vi "Enable Timers.vi"(0 "FPGA Ref":T6, 1 "Tank Data":T8 {"PS Actual (V):" format="%.2f"; "Temp1" format="%#_2g"; "Temp2" format="%#_2g"}, 2 "Tank CMDs":T7, 3 "App Config":T2={"Location"="", "Profiles Path"=path "", "Current Profile"="", "CA Number"="", "Cycles Completed"=0, "Controller Type:"=enum."Kuhnke", "Stagger Time (ms)"=0, "Tank 1 Fuel"="", "Tank 2 Fuel"="", "Serial Numbers"={"Position 1 SN"="", "Position 2 SN"="", "Poaition 3 SN"="", "Position 4 SN"="", "Position 5 SN"="", "Position 6 SN"=""}, "Pumps Present"={"Pump 1"=FALSE, "Pump 2"=FALSE, "Pump 3"=FALSE, "Pump 4"=FALSE, "Pump 5"=FALSE, "Pump 6"=FALSE}, "VoltCtrlRef"="", "VoltageSelect"=FALSE, "Watlow Present"=FALSE, "Temp 1"=0.0, "Temp 2"=0.0, "V_Run PI?"=FALSE, "Voltage Limits"={"V_Step"=1e-05, "V_CmdMax"=0.0, "V_CmdMin"=0.0}, "Voltage Far PI"={"V_FarSlew"=10.0, "V_FarKp"=0.0, "V_FarKi"=0.0}, "Voltage Mid PI"={"V_MidSlew"=10.0, "V_MidKp"=0.0, "V_MidKi"=0.0}, "Voltage Close PI"={"V_CloseSlew"=10.0, "V_CloseKp"=0.0, "V_CloseKi"=0.0}, "Voltage Scale"={"V_FFm"=0.0, "V_FFb"=0.0}, "Voltage Cutoffs"={"V_MidCutoff"=0.0, "V_CloseCutoff"=0.0}, "Pressure Scale"={"Pres_FFm"=1e-05, "Pres_FFb"=0.0}, "Temp Format"=0, "Temp Tolerance"=0.0, "Target Voltage"=0.0, "Target Pressure"=0.0, "Data Log Init"={"Data Path"=path "", "Data Log Rate (S/s)"=0, "AKLH Rate (Hours/S)"=0.0, "Sync Time Offset (min)"=0, "IP Last 3"=0, "WebDAV IP"=""}, "Email Handler IP"="", "ADC Check"=FALSE, "3 Pump Tank"=FALSE, "Cycle Threshold:"=3.0, "Cycle Pts to Avg:"=3, "Anomaly Threshold:"=3.0, "Normal Steps:"=3, "Step Threshold:"=3.0, "Network Drive IP"="", "Network Drive Password"="", "Bank 1 Offset"=0.0, "Bank 2 Offset"=0.0} {"Bank 2 Offset" min=0.0 max=999999.0 step=1.0; "Bank 1 Offset" min=0.0 max=999999.0 step=1.0; "Step Threshold:" min=0.0 max=999999.0 step=1.0; "Normal Steps:" max=999999 step=1; "Anomaly Threshold:" min=0.0 max=999999.0 step=1.0; "Cycle Pts to Avg:" max=999999 step=1; "Cycle Threshold:" min=0.0 max=999999.0 step=1.0}, 4 "Controller CMDs":dbl[](array[numeric]), 5 "Controller Config":T5, 6 "Run Profile":bool, 7 "Pumps Present":bool[](array[boolean])) -> (20 "In Spec":bool[](array[boolean]), 21 "Reset ADCs":bool)   [LabVIEW 2018]
uses:
  Controls/FPGA_Reference.ctl
  <vilib>/rvi/interface/nirviReadWriteControl/nirviReadWriteControl.xnode
  FPGA Bitfiles/LS_Durability_FPGA_9627.lvbitx
  <vilib>/rvi/errors/niLvFpgaMergeErrorWithErrorCode.vi
  <vilib>/rvi/errors/niLvFpgaAdjustHostInterfaceError.vi
  Controls/Tank Data.ctl
  Controls/Tank CMDs.ctl
  Type Defs/Controller Names.ctl
  Controls/Controller Config.ctl
  Type Defs/App Config.ctl
  Controls/Pump Data.ctl
  Data Logger/Data Log Init.ctl
panel:
  in  "Pump Data":T1={"Voltages"=[0.015201568603515625, 0.00335693359375, 0.003021240234375, 0.12260055541992188, 0.06085968017578125, 0.052234649658203125], "PumpCurrent"=[0.015201568603515625, 0.00335693359375, 0.003021240234375, 0.12260055541992188, 0.06085968017578125, 0.052234649658203125], "Speed"=[0.0, 0.0, 0.0, 0.0, 0.0, 0.0], "ControllerCurrent"=[0.015201568603515625, 0.00335693359375, 0.003021240234375, 0.12260055541992188, 0.06085968017578125, 0.052234649658203125], "Pressure"=[0.015201568603515625, 0.00335693359375, 0.003021240234375, 0.12260055541992188, 0.06085968017578125, 0.052234649658203125], "Flow"=[0.0, 0.0, 0.0, 0.125, 0.0625, 0.0625], "Elapsed Time (Display)"=[7.1, 7.1, 7.1, 458133.45, 458138.85000000003, 458126.75], "Avg Pressure"=0.0, "Avg Speed"=0.0, "Elapsed Time"=[4074.9003000000002, 4074.9003000000002, 4074.9003000000002, 4074.9003000000002, 4074.9003000000002, 4074.9003000000002]} {"Elapsed Time" format="%<%H:%M:%S>t"; "Elapsed Time (Display)" format="%<%H:%M:%S>t"; "Speed" format="%#_4f"; "ControllerCurrent" format="%#.1g"; "Pressure" format="%#.0f"; "Flow" format="%#.0f"; "PumpCurrent" format="%#.1g"; "Voltages" format="%#.0f"}
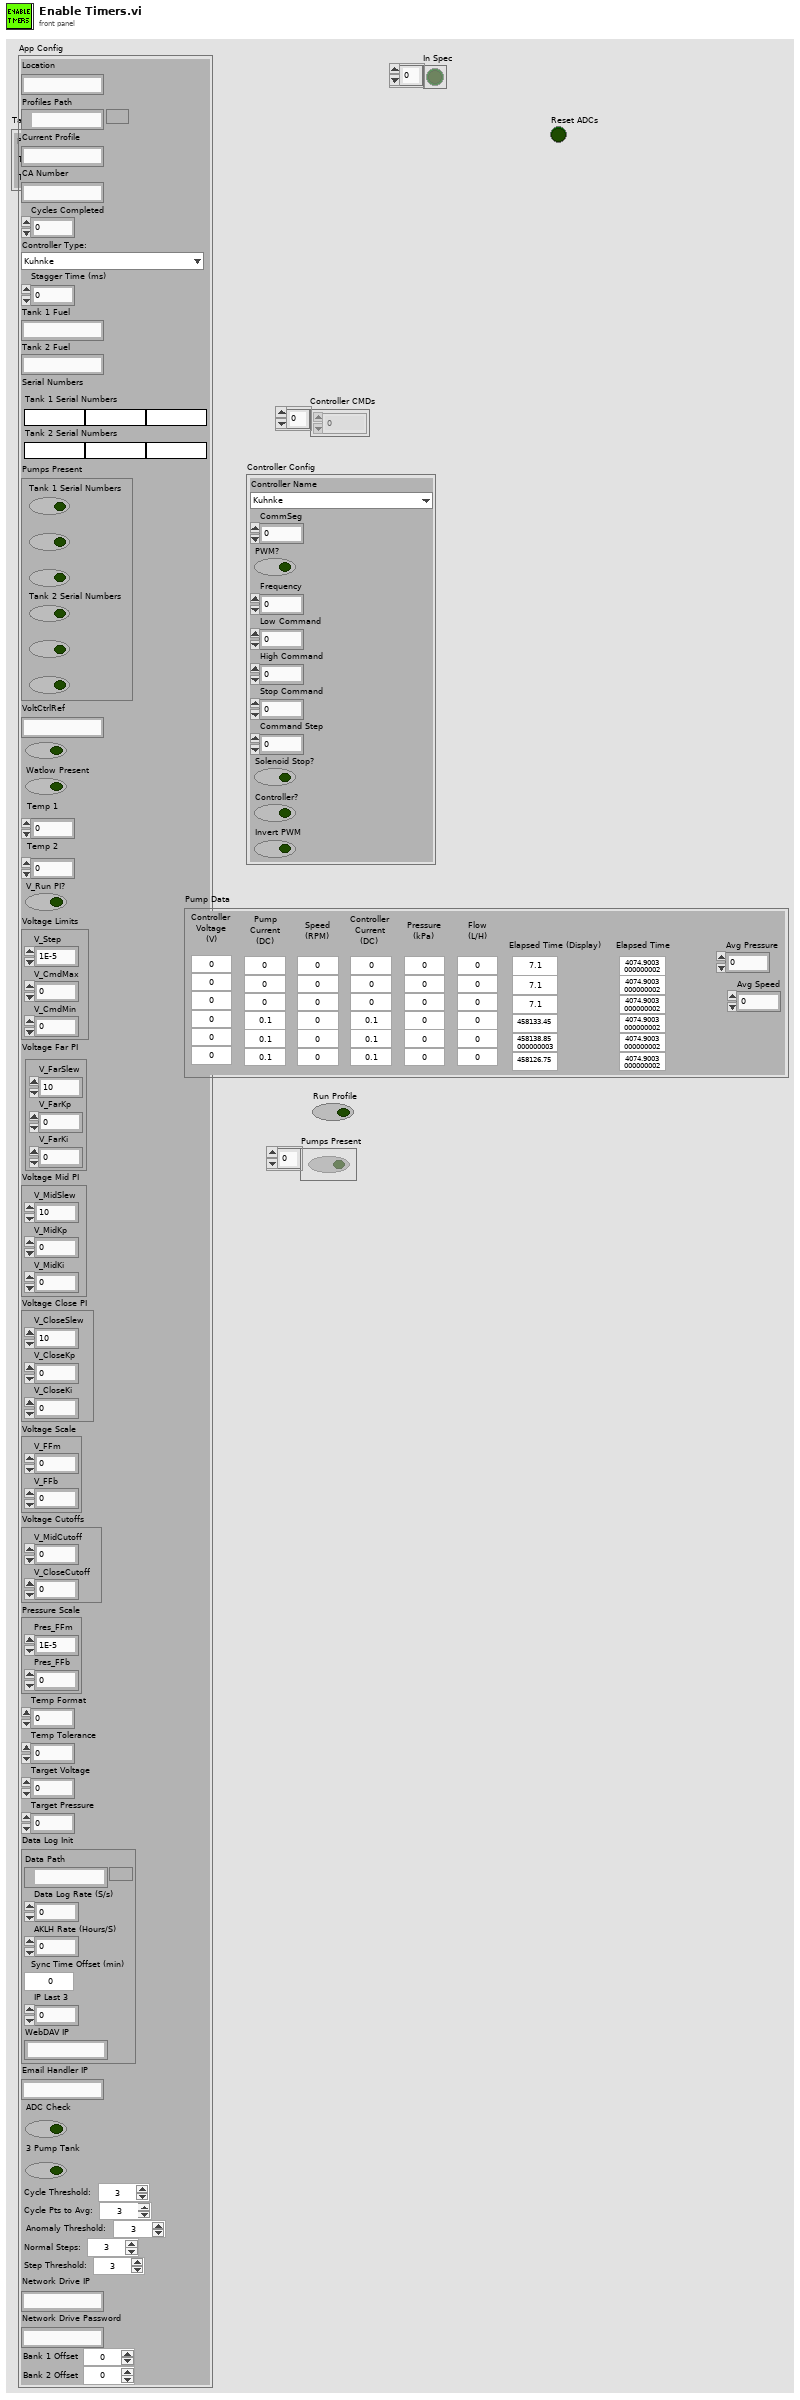
[diagram p1: front panel]
types:
  T1 = typedef "Pump Data.ctl" = cluster{"Voltages":dbl[], "PumpCurrent":dbl[], "Speed":dbl[], "ControllerCurrent":dbl[], "Pressure":dbl[], "Flow":dbl[], "Elapsed Time (Display)":dbl[], "Avg Pressure":dbl, "Avg Speed":dbl, "Elapsed Time":dbl[]}
  T2 = typedef "App Config.ctl" = cluster{"Location":string, "Profiles Path":path, "Current Profile":string, "CA Number":string, "Cycles Completed":u32, "Controller Type:":T3, "Stagger Time (ms)":i32, "Tank 1 Fuel":string, "Tank 2 Fuel":string, "Serial Numbers":cluster{"Position 1 SN":string, "Position 2 SN":string, "Poaition 3 SN":string, "Position 4 SN":string, "Position 5 SN":string, "Position 6 SN":string}, "Pumps Present":cluster{"Pump 1":bool, "Pump 2":bool, "Pump 3":bool, "Pump 4":bool, "Pump 5":bool, "Pump 6":bool}, "VoltCtrlRef":string, "VoltageSelect":bool, "Watlow Present":bool, "Temp 1":dbl, "Temp 2":dbl, "V_Run PI?":bool, "Voltage Limits":cluster{"V_Step":dbl, "V_CmdMax":dbl, "V_CmdMin":dbl}, "Voltage Far PI":cluster{"V_FarSlew":dbl, "V_FarKp":dbl, "V_FarKi":dbl}, "Voltage Mid PI":cluster{"V_MidSlew":dbl, "V_MidKp":dbl, "V_MidKi":dbl}, "Voltage Close PI":cluster{"V_CloseSlew":dbl, "V_CloseKp":dbl, "V_CloseKi":dbl}, "Voltage Scale":cluster{"V_FFm":dbl, "V_FFb":dbl}, "Voltage Cutoffs":cluster{"V_MidCutoff":dbl, "V_CloseCutoff":dbl}, "Pressure Scale":cluster{"Pres_FFm":dbl, "Pres_FFb":dbl}, "Temp Format":i32, "Temp Tolerance":dbl, "Target Voltage":dbl, "Target Pressure":dbl, "Data Log Init":T4, "Email Handler IP":string, "ADC Check":bool, "3 Pump Tank":bool, "Cycle Threshold:":dbl, "Cycle Pts to Avg:":i32, "Anomaly Threshold:":dbl, "Normal Steps:":u32, "Step Threshold:":dbl, "Network Drive IP":string, "Network Drive Password":string, "Bank 1 Offset":dbl, "Bank 2 Offset":dbl}
  T3 = typedef "Controller Names.ctl" = enum16{"Kuhnke", "Helbako BLDC", "Conti", "Hella BLDC OL PWM", "Hella BLDC Turbine OL PWM", "Hella BLDC Pressure", "Helbako (old)", "TI PWM", "PSA", "Hella Gas", "Hella Diesel", "8 Comm", "10 Comm", "8 Comm Hella", "10 Comm Hella", "8 Comm Omron", "10 Comm Omron", "8 Comm Nissan", "10 Comm Nissan"}
  T4 = typedef "Data Log Init.ctl" = cluster{"Data Path":path, "Data Log Rate (S/s)":u32, "AKLH Rate (Hours/S)":dbl, "Sync Time Offset (min)":i32, "IP Last 3":i32, "WebDAV IP":string}
  T5 = typedef "Controller Config.ctl" = cluster{"Controller Name":T3, "CommSeg":i32, "PWM?":bool, "Frequency":i32, "Low Command":dbl, "High Command":dbl, "Stop Command":dbl, "Command Step":dbl, "Solenoid Stop?":bool, "Controller?":bool, "Invert PWM":bool}
  T6 = typedef "FPGA_Reference.ctl" = refnum<k20>
  T7 = typedef "Tank CMDs.ctl" = cluster{"PS CMD":dbl, "Press CMD":dbl, "Temp 1 CMD":dbl, "Temp 2 CMD":dbl}
  T8 = typedef "Tank Data.ctl" = cluster{"PS Actual (V):":dbl, "Temp1":dbl, "Temp2":dbl}
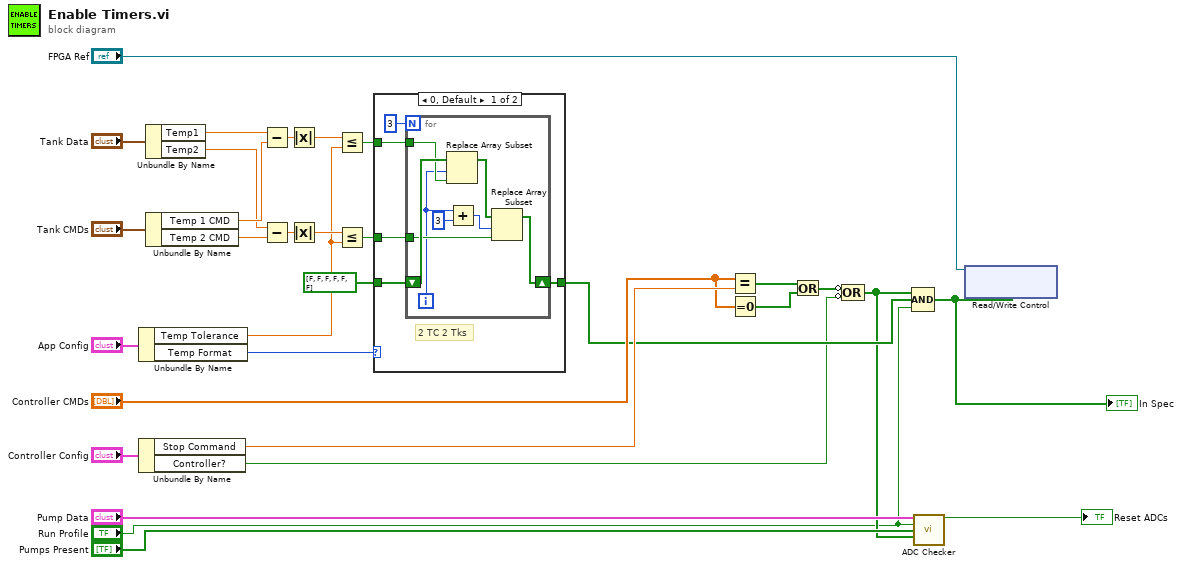
[diagram p0: block diagram]
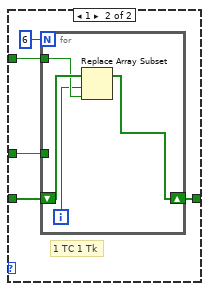
[diagram p2: hidden frame]
diagram:
  n1 = Unbundle By Name("App Config") -> ("Temp Tolerance"=w8:dbl, "Temp Format"=w7:i32)
  n2 = Unbundle By Name("Controller Config") -> ("Stop Command"=w12:dbl, "Controller?"=w6:bool)
  n3 = Unbundle By Name("Tank Data") -> ("Temp1"=w25:dbl, "Temp2"=w26:dbl)
  n4 = Unbundle By Name("Tank CMDs") -> ("Temp 1 CMD"=w27:dbl, "Temp 2 CMD"=w28:dbl)
  n5 = Subtract(x=w25, y=w27) -> (x-y=w24:dbl)
  n6 = Subtract(x=w26, y=w28) -> (x-y=w23:dbl)
  n7 = Absolute Value(x=w24) -> (abs(x)=w22:dbl)
  n8 = Absolute Value(x=w23) -> (abs(x)=w21:dbl)
  n9 = Less Or Equal?(x=w22, y=w8) -> (x <= y?=w29:bool)
  n10 = Less Or Equal?(x=w21, y=w8) -> (x <= y?=w30:bool)
  n11 = case shown="0, Default" w7 {
    tunnel: w29 -> [w34 w47]
    tunnel: w30 -> [w35 w48]
    tunnel: bool[] [FALSE, FALSE, FALSE, FALSE, FALSE, FALSE] -> [w36 w49]
    tunnel: [w33 w46] -> w10
    frame 0, Default {
      # "2 TC 2 Tks"
      n12 = for {
        N: 3 -> [_]
        shift-right: [w40] -> w33
        shift-left: w36 -> [w44]
        tunnel: w35 -> [w41]
        tunnel: w34 -> [w42]
        i -> [w38]
        n13 = Replace Array Subset(array=w44, new element=w42, index=w38) -> (w43:bool[])
        n14 = Add(x=w38, y=3) -> (x+y=w39:i32)
        n15 = Replace Array Subset(array=w43, new element=w41, index=w39) -> (w40:bool[])
      }
    }
    frame 1 {
      # "1 TC 1 Tk"
      n16 = for {
        N: 6 -> [_]
        shift-right: [w50] -> w46
        shift-left: w49 -> [w53]
        tunnel: w48 -> [_]
        tunnel: w47 -> [w52]
        i -> [w51]
        n17 = Replace Array Subset(array=w53, new element=w52, index=w51) -> (w50:bool[])
      }
    }
  }
  n18 = Equal?(x="Controller CMDs", y=w12) -> (x = y?=w18:bool[])
  n19 = Equal To 0?(x="Controller CMDs") -> (x = 0?=w15:bool[])
  n20 = Or(x=w18, y=w15) -> (x .or. y?=w16:bool[])
  n21 = Compound Arithmetic op=OR(invert w16, invert w6) -> (w3:bool[])
  n22 = Compound Arithmetic op=AND(w3, w10, "Run Profile") -> (w17:bool[])
  "In Spec" <- w17
  n23 = call "ADC Checker.vi"("Pump Data"="Pump Data", "Run Profile"="Run Profile", "Pumps Present"="Pumps Present", "Not Stopped"=w3) -> ("Reset ADCs"=→"Reset ADCs":bool)  [unwired: 11 in]
  n24 = xnode "Read/Write Control"("FPGA VI Reference In"="FPGA Ref", "Enable Timers"=w17) -> ()  [unwired: 1 in, 2 out]
